vi "PH_BeamlineController.set current Value of Target Elements.vi"(0 "VI in":refnum<vi>, 5 "error in (no error)":errorcluster) -> (14 "VI out":refnum<vi>, 19 "error out":errorcluster)   [LabVIEW 2014, in "PH_BeamlineController.lvlib"]
uses:
  PH_BeamlineController.lvlib
  PH_Beamline_Chief/PH_Beamline_Chief.Section.ctl
  PH_BeamlineInformation/PH_BeamlineInformation.lvlib
  PH_Beamline_Chief/PH_Beamline_Chief.lvlib
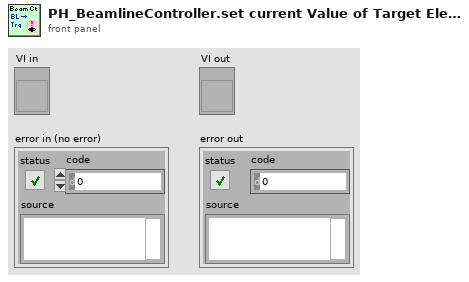
[diagram p1: front panel]
types:
  T1 = typedef "PH_BeamlineController.lvlib/PH_BeamlineController.i attribute.ctl" = cluster{"Vacuum Exp LB":cluster{"Channel":string, "Limit [mbar]":dbl, "Pressure [mbar]":dbl, "GUI Ref":refnum<vi>}, "Sources":T2[], "PA DP Targets":T4[], "Path":cluster{"Source":T3, "PA DP Target":T5, "Target":T6}, "Targets":cluster{"Name":T6, "GUI Ref":refnum<vi>, "Current State":bool, "Wanted State":bool, "Enabled":bool}[], "Status Tags":cluster{"Name":string, "Status":T7}[], "special GUI Refs":T8}
  T2 = typedef "PH_BeamlineController.lvlib/PH_BeamlineController.Source Attributes.ctl" = cluster{"Name":T3, "GUI Ref":refnum<vi>, "Current State":bool, "Wanted State":bool}
  T3 = typedef "PH_BeamlineController.lvlib/PH_BeamlineController.Sources.ctl" = enum16{"None", "YLF", "fs-Frontend", "ns-Frontend", "YLF and ns-Frontend", "fs- and ns-Frontend"}
  T4 = typedef "PH_BeamlineController.lvlib/PH_BeamlineController.PA DP Target Attributes.ctl" = cluster{"Name":T5, "GUI Ref":refnum<vi>, "Current State":bool, "Wanted State":bool, "Enabled":bool}
  T5 = typedef "PH_BeamlineController.lvlib/PH_BeamlineController.PA DP Targets.ctl" = enum16{"None", "Dump PA Delayed Beam", "Dump PA Undelayed Beam", "Dumps PA Delayed and Undelayed Beam"}
  T6 = typedef "PH_BeamlineController.lvlib/PH_BeamlineController.Targets.ctl" = enum16{"None", "PreAmp", "Dump Exp Laserlab", "Exp Laserlab", "Calorimeter", "Dump Exp Laserbay", "Exp Laserbay", "Dump Exp Z6", "Exp Z6"}
  T7 = typedef "PH_StatusHandler.lvlib/PH_StatusHandler.Status.ctl" = i16
  T8 = typedef "PH_BeamlineController.lvlib/PH_BeamlineController.special GUI Refs.ctl" = cluster{"PA-Backreflection-Meas":refnum<vi>, "fs_Synchrolock_Watch":refnum<vi>}
  T9 = cluster{"Name":T6, "GUI Ref":refnum<vi>, "Current State":bool, "Wanted State":bool, "Enabled":bool}[]
  T10 = typedef "PH_Beamline_Chief.lvlib/PH_Beamline_Chief.Section.ctl" = enum16{"None", "YLF", "fs", "fs-YLF", "ns", "PA-Input", "PA-Undelay", "PA-Delay", "PA-before-Bypass", "PA", "PA-Bypass", "PA-Exit", "PA-LL", "LL", "PA-MA", "MA-Exit", "MA-Z6", "Z6", "MA-LB", "LB-TB2", "LB-TB3"}
  T11 = typedef "PH_BeamlineController.lvlib/PH_BeamlineController.Target Attributes.ctl" = cluster{"Name":T6, "GUI Ref":refnum<vi>, "Current State":bool, "Wanted State":bool, "Enabled":bool}
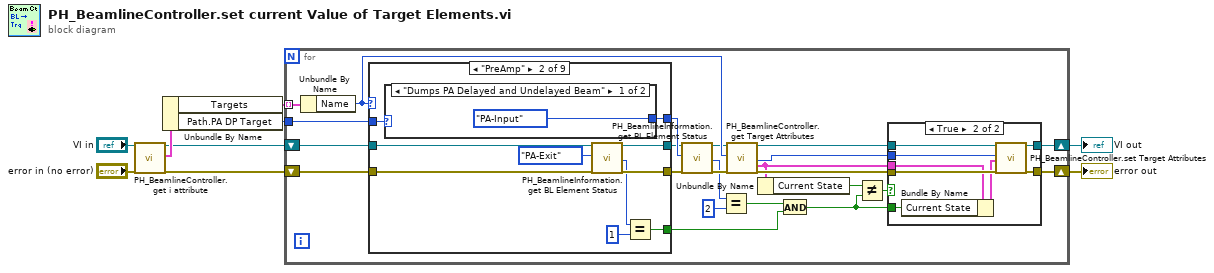
[diagram p0: block diagram]
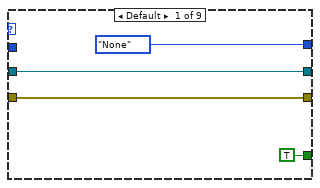
[diagram p2: hidden frame]
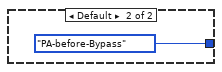
[diagram p3: hidden frame]
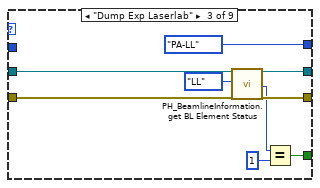
[diagram p4: hidden frame]
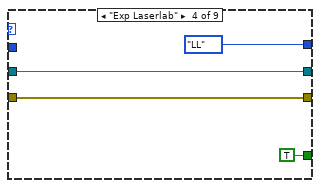
[diagram p5: hidden frame]
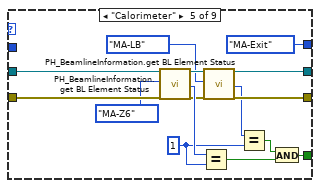
[diagram p6: hidden frame]
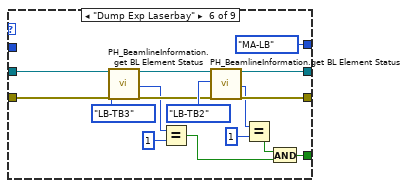
[diagram p7: hidden frame]
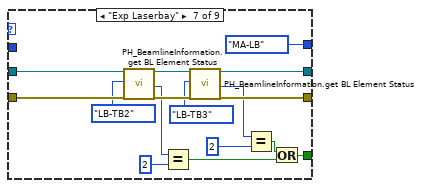
[diagram p8: hidden frame]
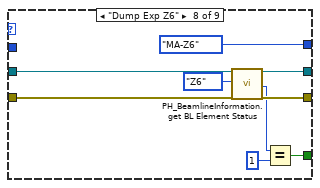
[diagram p9: hidden frame]
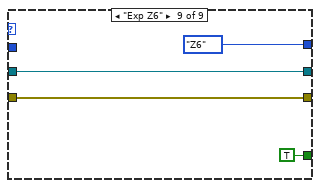
[diagram p10: hidden frame]
diagram:
  n1 = call "PH_BeamlineController.get i attribute.vi"("i ref in"="VI in", "error in (no error)"="error in (no error)") -> ("i ref out"=w5:refnum<vi>, "i attribute"=w9:T1, "error out"=w4:errorcluster)  [unwired: 15 in]
  n2 = Unbundle By Name(w9) -> ("Targets"=w6:T9, "Path.PA DP Target"=w1:T5)
  n3 = for {
    shift-right: [w31] -> w8
    shift-left: w4 -> [w14]
    shift-right: [w29] -> w7
    shift-left: w5 -> [w16]
    tunnel: w6 -> [w27] mode=indexing
    tunnel: w1 -> [w10]
    n4 = Unbundle By Name(w27) -> ("Name"=w23:T6)
    n5 = case shown="\"PreAmp\"" w23 {
      tunnel: [PH_Beamline_Chief.Section."None" ("Beamline Element") w46 PH_Beamline_Chief.Section."PA-LL" ("Beamline Element") PH_Beamline_Chief.Section."LL" ("Beamline Element") PH_Beamline_Chief.Section."MA-Exit" ("Beamline Element") PH_Beamline_Chief.Section."MA-LB" ("Beamline Element") PH_Beamline_Chief.Section."MA-LB" ("Beamline Element") PH_Beamline_Chief.Section."MA-Z6" ("Beamline Element") PH_Beamline_Chief.Section."Z6" ("Beamline Element")] -> w20
      tunnel: w16 -> [w35 w43 w54 w60 w74 w85 w105 w114 w120]
      tunnel: [w35 w42 w53 w60 w70 w90 w107 w113 w120] -> w15
      tunnel: w14 -> [w34 w45 w56 w59 w75 w83 w103 w116 w119]
      tunnel: [w34 w44 w55 w59 w68 w91 w106 w115 w119] -> w13
      tunnel: [TRUE w38 w49 TRUE w62 w79 w95 w109 TRUE] -> w11
      tunnel: w10 -> [_ w37 _ _ _ _ _ _ _]
      frame Default {
      }
      frame "PreAmp" {
        n6 = case shown="\"Dumps PA Delayed and Undelayed Beam\"" w37 {
          tunnel: [PH_Beamline_Chief.Section."PA-Input" ("Beamline Element") PH_Beamline_Chief.Section."PA-before-Bypass" ("Beamline Element")] -> w46
          frame "Dumps PA Delayed and Undelayed Beam" {
          }
          frame Default {
          }
        }
        n7 = call "PH_BeamlineInformation.get BL Element Status.vi"("VI in"=w43, "Beamline Element"=PH_Beamline_Chief.Section."PA-Exit", "error in (no error)"=w45) -> ("VI out"=w42:refnum<vi>, "Status"=w39:i32, "error out"=w44:errorcluster)  [unwired: 14 in]
        n8 = Equal?(x=w39, y=1) -> (x = y?=w38:bool)
      }
      frame "Dump Exp Laserlab" {
        n9 = call "PH_BeamlineInformation.get BL Element Status.vi"("VI in"=w54, "Beamline Element"=PH_Beamline_Chief.Section."LL", "error in (no error)"=w56) -> ("VI out"=w53:refnum<vi>, "Status"=w50:i32, "error out"=w55:errorcluster)  [unwired: 14 in]
        n10 = Equal?(x=w50, y=1) -> (x = y?=w49:bool)
      }
      frame "Exp Laserlab" {
      }
      frame "Calorimeter" {
        w66 = 1 ("y")
        n11 = call "PH_BeamlineInformation.get BL Element Status.vi"("VI in"=w74, "Beamline Element"=PH_Beamline_Chief.Section."MA-Z6", "error in (no error)"=w75) -> ("VI out"=w71:refnum<vi>, "Status"=w72:i32, "error out"=w69:errorcluster)  [unwired: 14 in]
        n12 = Equal?(x=w72, y=w66) -> (x = y?=w63:bool)
        n13 = call "PH_BeamlineInformation.get BL Element Status.vi"("VI in"=w71, "Beamline Element"=PH_Beamline_Chief.Section."MA-LB", "error in (no error)"=w69) -> ("VI out"=w70:refnum<vi>, "Status"=w67:i32, "error out"=w68:errorcluster)  [unwired: 14 in]
        n14 = Equal?(x=w67, y=w66) -> (x = y?=w64:bool)
        n15 = And(x=w64, y=w63) -> (x .and. y?=w62:bool)
      }
      frame "Dump Exp Laserbay" {
        n16 = call "PH_BeamlineInformation.get BL Element Status.vi"("VI in"=w85, "Beamline Element"=PH_Beamline_Chief.Section."LB-TB3", "error in (no error)"=w83) -> ("VI out"=w84:refnum<vi>, "Status"=w80:i32, "error out"=w82:errorcluster)  [unwired: 14 in]
        n17 = Equal?(x=w80, y=1) -> (x = y?=w77:bool)
        n18 = call "PH_BeamlineInformation.get BL Element Status.vi"("VI in"=w84, "Beamline Element"=PH_Beamline_Chief.Section."LB-TB2", "error in (no error)"=w82) -> ("VI out"=w90:refnum<vi>, "Status"=w87:i32, "error out"=w91:errorcluster)  [unwired: 14 in]
        n19 = Equal?(x=w87, y=1) -> (x = y?=w78:bool)
        n20 = And(x=w78, y=w77) -> (x .and. y?=w79:bool)
      }
      frame "Exp Laserbay" {
        n21 = call "PH_BeamlineInformation.get BL Element Status.vi"("VI in"=w105, "Beamline Element"=PH_Beamline_Chief.Section."LB-TB2", "error in (no error)"=w103) -> ("VI out"=w104:refnum<vi>, "Status"=w99:i32, "error out"=w102:errorcluster)  [unwired: 14 in]
        n22 = Equal?(x=w99, y=2) -> (x = y?=w93:bool)
        n23 = call "PH_BeamlineInformation.get BL Element Status.vi"("VI in"=w104, "Beamline Element"=PH_Beamline_Chief.Section."LB-TB3", "error in (no error)"=w102) -> ("VI out"=w107:refnum<vi>, "Status"=w97:i32, "error out"=w106:errorcluster)  [unwired: 14 in]
        n24 = Equal?(x=w97, y=2) -> (x = y?=w94:bool)
        n25 = Or(x=w94, y=w93) -> (x .or. y?=w95:bool)
      }
      frame "Dump Exp Z6" {
        n26 = call "PH_BeamlineInformation.get BL Element Status.vi"("VI in"=w114, "Beamline Element"=PH_Beamline_Chief.Section."Z6", "error in (no error)"=w116) -> ("VI out"=w113:refnum<vi>, "Status"=w110:i32, "error out"=w115:errorcluster)  [unwired: 14 in]
        n27 = Equal?(x=w110, y=1) -> (x = y?=w109:bool)
      }
      frame "Exp Z6" {
      }
    }
    n28 = call "PH_BeamlineInformation.get BL Element Status.vi"("VI in"=w15, "Beamline Element"=w20, "error in (no error)"=w13) -> ("VI out"=w22:refnum<vi>, "Status"=w19:i32, "error out"=w21:errorcluster)  [unwired: 14 in]
    n29 = Equal?(x=w19, y=2) -> (x = y?=w17:bool)
    n30 = call "PH_BeamlineController.get Target Attributes.vi"("VI in"=w22, "Target"=w23, "error in (no error)"=w21) -> ("VI out"=w30:refnum<vi>, "Target Index"=w28:i32, "Target Attributes"=w26:T11, "error out"=w32:errorcluster)  [unwired: 13 in]
    n31 = Unbundle By Name(w26) -> ("Current State"=w25:bool)
    n32 = And(x=w17, y=w11) -> (x .and. y?=w12:bool)
    n33 = Not Equal?(x=w25, y=w12) -> (x != y?=w24:bool)
    n34 = case shown="True" w24 {
      tunnel: w32 -> [w122 w131]
      tunnel: [w122 w130] -> w31
      tunnel: w30 -> [w123 w129]
      tunnel: [w123 w128] -> w29
      tunnel: w28 -> [_ w127]
      tunnel: w26 -> [_ w125]
      tunnel: w12 -> [_ w124]
      frame False {
      }
      frame True {
        n35 = Bundle By Name(cluster=w125, "Current State"=w124) -> (w126:T11)
        n36 = call "PH_BeamlineController.set Target Attributes.vi"("VI in"=w129, "Target Index"=w127, "Changed Target Attributes"=w126, "error in (no error)"=w131) -> ("VI out"=w128:refnum<vi>, "error out"=w130:errorcluster)  [unwired: 14 in]
      }
    }
  }
  "VI out" <- w7
  "error out" <- w8
